vi "Base example.vi"(10 "Color icon in":T1, 11 "BW icon in":T1) -> (0 "error out":errorcluster, 2 "Color icon out":T1, 3 "BW icon out":T1)   [LabVIEW 2021, in "Base example.lvlib"]
uses:
  <vilib>/picture/picture.llb/imagedata.ctl
  Base example.lvlib
panel:
  in  "Code":i32 caption="Set to 43 to signal that user cancelled"
  # "Save this VI after modifying \nthe default values of the control"
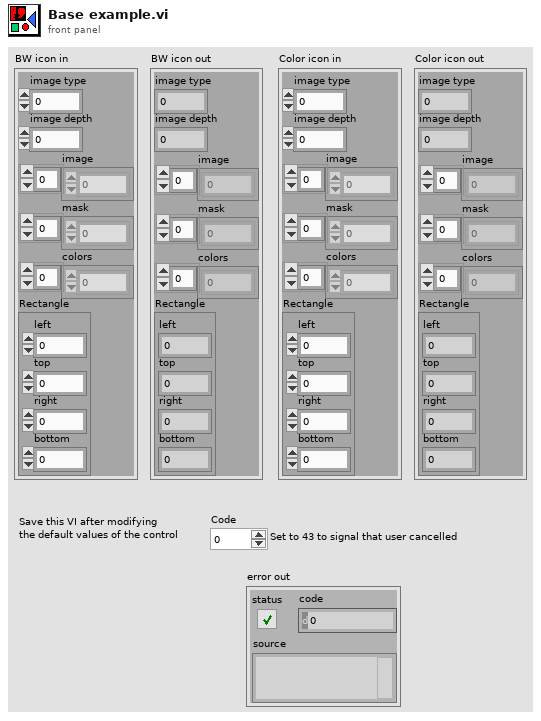
[diagram p1: front panel]
types:
  T1 = typedef "imagedata.ctl" = cluster{"image type":i32, "image depth":i32, "image":u8[], "mask":u8[], "colors":u32[], "Rectangle":cluster{"left":i16, "top":i16, "right":i16, "bottom":i16}}
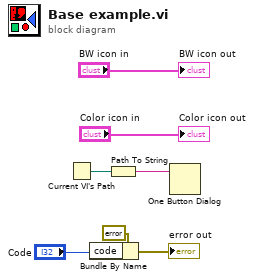
[diagram p0: block diagram]
diagram:
  n1 = Current VI's Path() -> (path=w2:path)
  n2 = Bundle By Name(cluster=errorcluster {"status"=FALSE, "code"=0, "source"=""} ("error out"), "code"="Code") -> (→"error out":errorcluster)
  n3 = Path To String(path=w2) -> (string=w1:string)
  n4 = One Button Dialog(message=w1) -> ()  [unwired: 1 in, 1 out]
  "BW icon out" <- "BW icon in"
  "Color icon out" <- "Color icon in"
